vi "Main.vi"() -> ()   [LabVIEW 2020]
doc: "This Continuous Measurement sample project is based on the Queued Message Handler template.\n\nThe Event Handling Loop generates messages based on user interface actions.\n\nThe Message Handling Loop processes messages generated by the Event Handling Loop, or by other messages. There are also Acquisition and Logging message handling loop subVIs, and a chart updating loop.\n\n20190717\nIntégration de la classe Image acquisition \nIntégration de la classe CAMERA_IDS\n\nModification de la FIFO, elle est limitée à 4096 image ; \nacquisition se fait en fonction de la fréquence trame ; \naprès la sauvegarde des images on repasse à l'état acquisition. \n\n20170719\nIntegration de la classe camera PCO.\nLa fonction RUN est deplace dans getImage, pour mettre la camera dans l etat Run on verifie si les deux booleens Buffer0 et Buffer1 sont a Vrai. Start met ces deux booleens a Vrai ensuite l4un est le complement de l autre.\nModification de l affichage de Sav\nModification de la boite de dialogue maintenant on affiche les anciennes valeurs\nModification de init et exit : \nOn fait un seul init ;\non arrete pas la camera avec Stop mais avec Exit.\nAcquisition au format U16, sauvegarde FITS au format U16\nOn ralentit l affichage des images a 10 Hz> \nTest ROI 960x960 Trigger Externe 100 Hz on arrive a acquerir des cubes de 1024 images."
uses:
  UI Data.ctl
  SETTING/Settings.ctl
  LOGGING/Logging Configuration.ctl
  ACQUISITION/HardwareConfiguration.ctl
  CLASS/Image Acquisition Class/Camera.lvclass
  MIRROR/mirror.lvclass
  SETTING/data_Display.ctl
  SETTING/data_Queue.ctl
  CLASS/simuCalc Class/simuCalc.lvclass
  D:/USERS/MONTRI/BABYDOL/LABVIEW/EXEMPLE_ARCHITECTURE/acquImageCont_Sav2FITS/CLASS/Image Acquisition Class/Camera.lvclass
  ACQUISITION/Acquisition.lvlib
  LOGGING/Logging.lvlib
  SETTING/Settings.lvlib
  USER_EVENT/User Event - Stop.lvlib
  MESSAGE_QUEUE/Message Queue.lvlib
panel:
  in  "milliseconds to wait":u32=20
  out "vectCom":cluster{"tabCdG[0]":sgl, "tabCdG[1]":sgl}(graph)
  in  "loop gain (0)":dbl min=0.0 max=1.0 step=0.01
  in  "closeLoop":bool
  in  "CenterOfGravity":bool
  out "tabCdG":cluster{"tabCdG[0]":sgl, "tabCdG[1]":sgl}(graph)
  in  "threshold":bool
  in  "thresholdValue (85)":dbl
  in  "Settings":bool
  in  "Save":bool
  in  "Background":bool
  in  "LUT":bool
  in  "subtract Backgound":bool
  out "Data":sgl[][](graph)
  out "Status":string
  in  "Start":bool
  in  "Stop":bool
  in  "Exit":bool
  # "Continuous Image Acquisition"
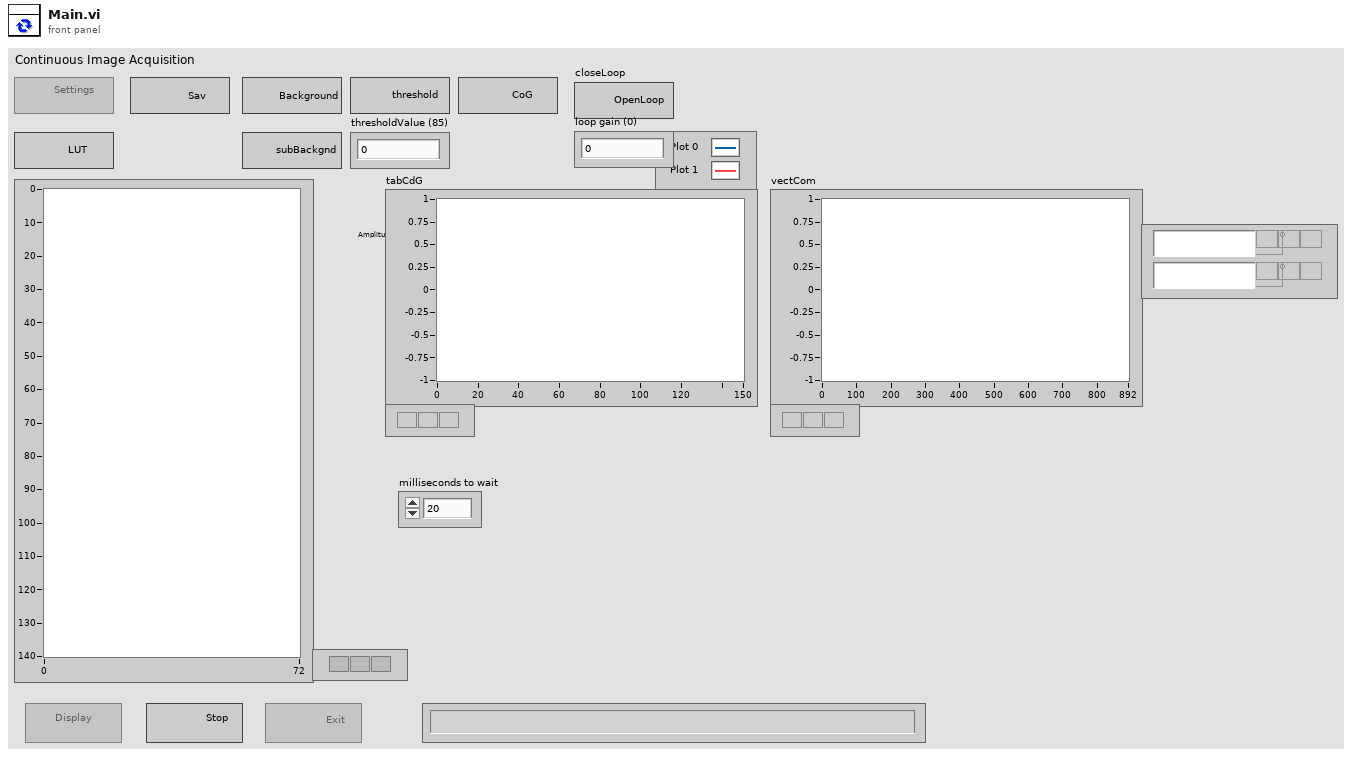
[diagram p1: front panel]
types:
  T1 = typedef "data_Queue.ctl" = cluster{"tabIma":u16[][], "tabCdG":sgl[], "vectCom":sgl[]}
  T2 = typedef "data_Display.ctl" = cluster{"tabIma":sgl[][], "tabCdG":sgl[], "vectCom":sgl[]}
  T3 = typedef "Settings.lvlib/Settings.ctl" = cluster{"Logging Configuration":T4, "camera":T5}
  T4 = typedef "Logging.lvlib/Logging Configuration.ctl" = cluster{"Log File Base Path":path, "NbrIma":i32}
  T5 = typedef "Acquisition.lvlib/HardwareConfiguration.ctl" = cluster{"Camera.lvclass":refnum<class "Camera.lvclass">, "InClusTiming 2":cluster{"Pixelclock":i32, "Exposure":dbl, "ExposureTimeBase":u16, "Framerate":dbl, "TriggerMode":u16}, "ROI":cluster{"PosX":i32, "PosY":i32, "Width":i32, "Height":i32}, "File Path Control":path, "mirror.lvclass":refnum<class "mirror.lvclass">}
  T6 = typedef "UI Data.ctl" = cluster{"Start Ref":refnum<vi>, "Save Ref":refnum<vi>, "Background":refnum<vi>, "Stop Ref":refnum<vi>, "Settings Ref":refnum<vi>, "Exit Ref":refnum<vi>, "Status Ref":refnum<vi>, "Data Ref":refnum<vi>}
  T7 = typedef "Message Queue.lvlib/All Message Queues.ctl" = cluster{"UI":refnum<queue>, "Acquisition":refnum<queue>, "Logging":refnum<queue>}
  T8 = cluster{"threshold":bool, "thresholdValue (0)":dbl}
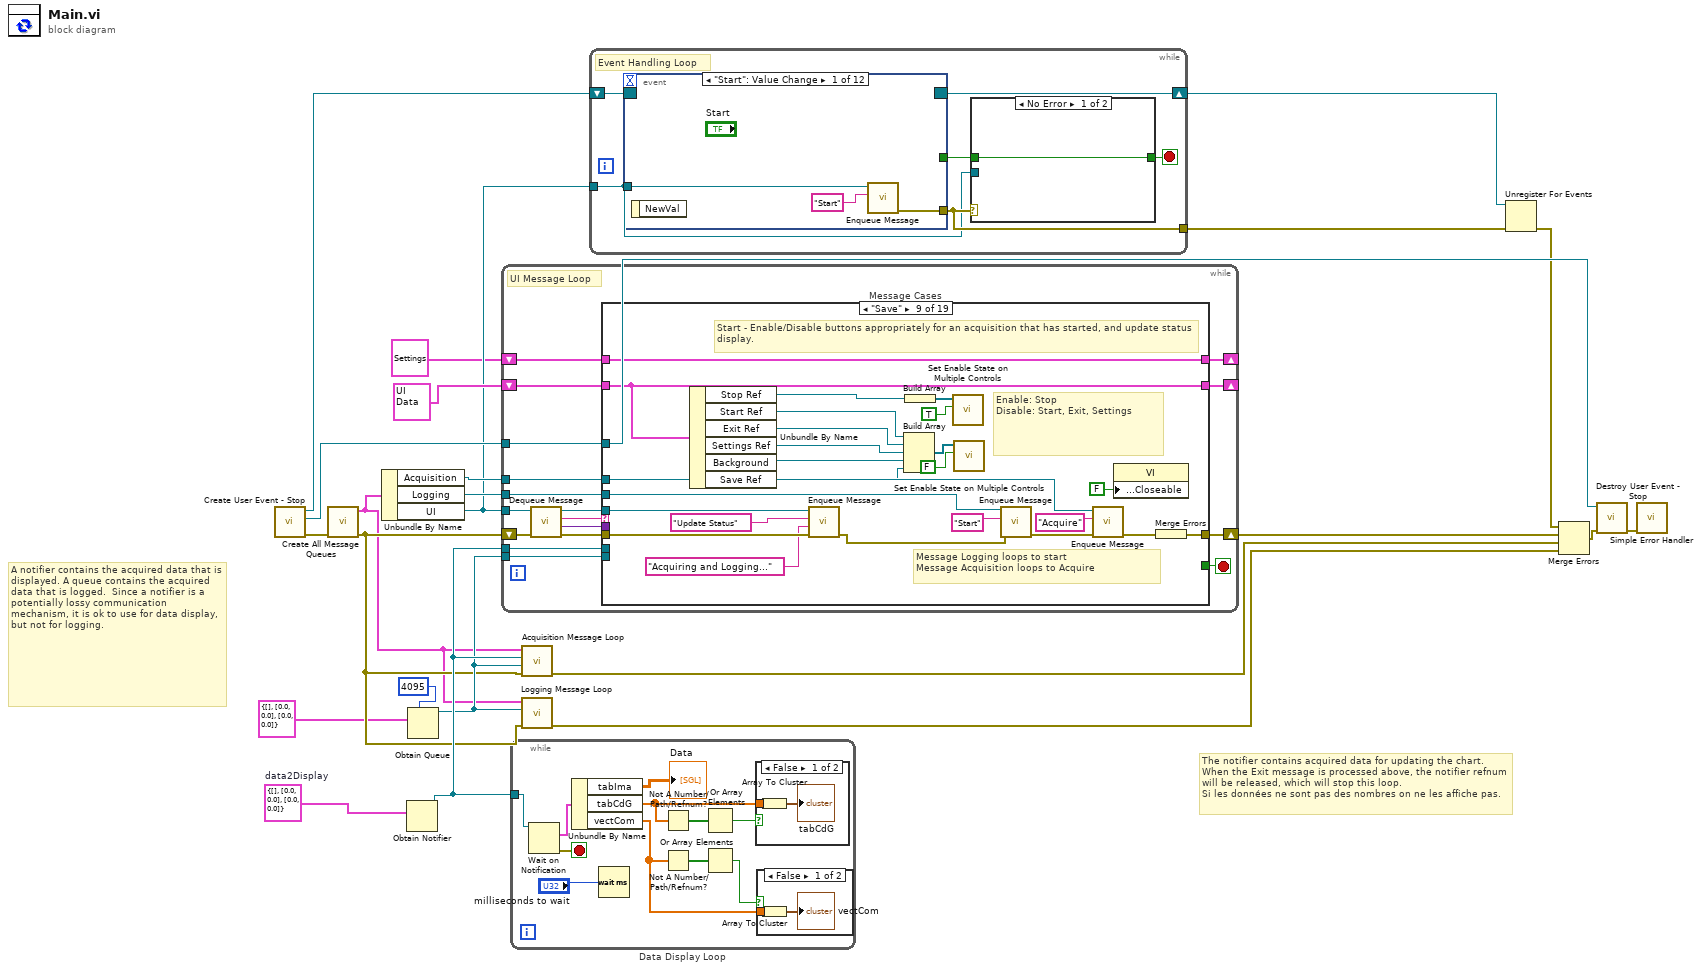
[diagram p0: block diagram]
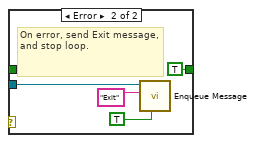
[diagram p4: hidden frame]
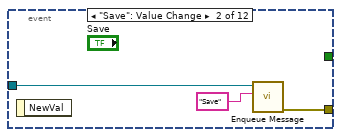
[diagram p5: hidden frame]
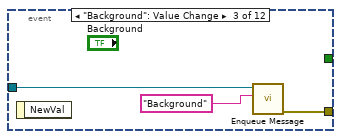
[diagram p6: hidden frame]
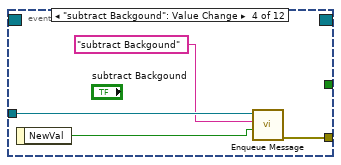
[diagram p7: hidden frame]
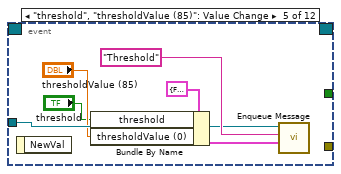
[diagram p8: hidden frame]
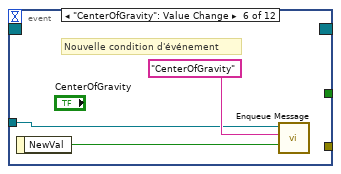
[diagram p9: hidden frame]
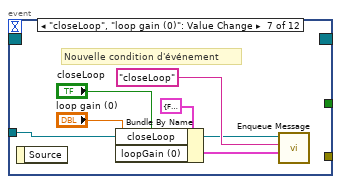
[diagram p10: hidden frame]
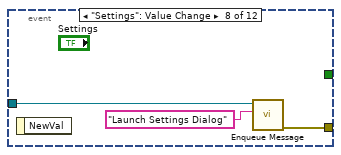
[diagram p11: hidden frame]
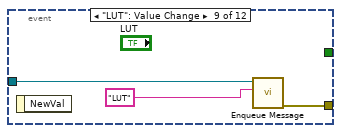
[diagram p12: hidden frame]
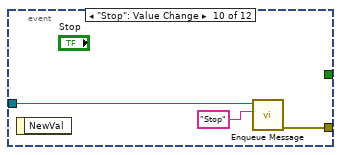
[diagram p13: hidden frame]
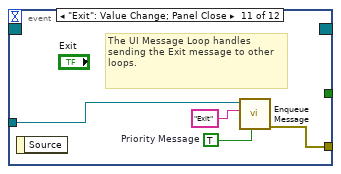
[diagram p14: hidden frame]
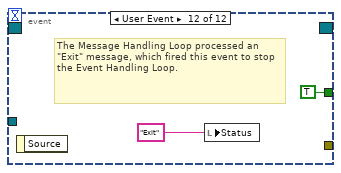
[diagram p15: hidden frame]
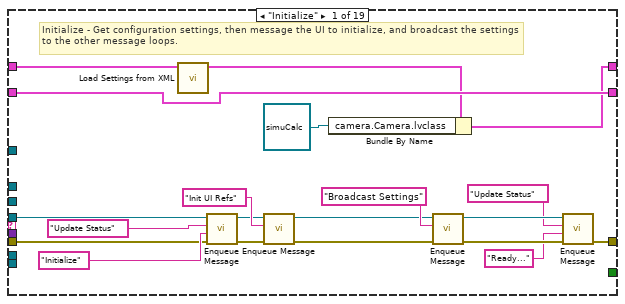
[diagram p16: hidden frame]
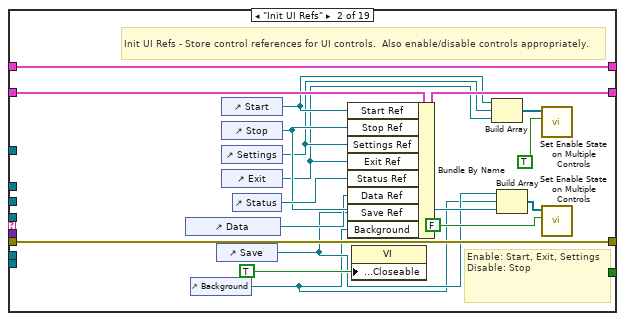
[diagram p17: hidden frame]
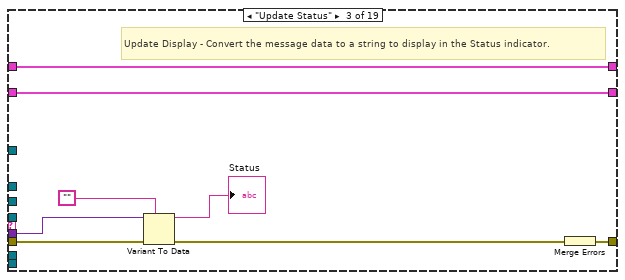
[diagram p18: hidden frame]
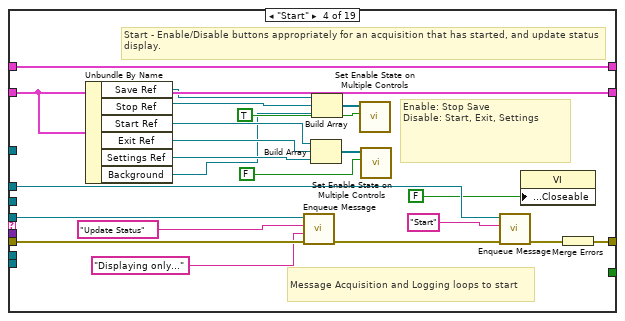
[diagram p19: hidden frame]
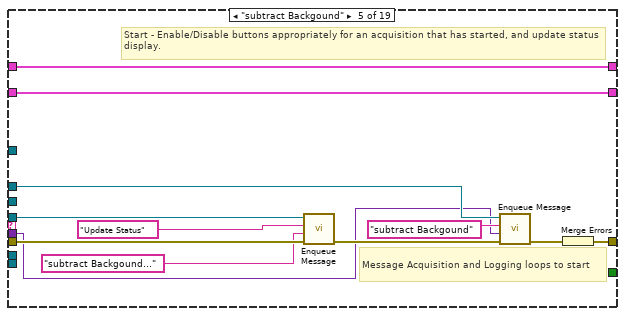
[diagram p20: hidden frame]
diagram:
  w2 = T2 {"tabIma"=[], "tabCdG"=[0.0, 0.0], "vectCom"=[0.0, 0.0]}  # data2Display
  # "A notifier contains the acquired data that is displayed. A queue contains the acquired data that is logged.  Since a notifier is a potentially lossy communication mechanism, it is ok to use for data display, but not for logging."
  # "The notifier contains acquired data for updating the chart. When the Exit message is processed above, the notifier refnum will be released, which will stop this loop.\nSi les données ne sont pas des nombres on ne les affiche pas."
  n1 = call "Create User Event - Stop.vi"() -> ("error out"=w17:errorcluster, "User Event - Stop"=w19:refnum<user-event>, "Stop Event Registration Refnum"=w20:refnum<event-registration>)  [unwired: 9 in]
  n2 = call "Create All Message Queues.vi"("error in (no error)"=w17) -> ("error out"=w4:errorcluster, "Message Queues out"=w3:T7)  [unwired: 9 in]
  n3 = Unbundle By Name(w3) -> ("Acquisition"=w12:refnum<queue>, "Logging"=w11:refnum<queue>, "UI"=w10:refnum<queue>)
  n4 = Obtain Notifier(notification data type=w2) -> (notifier out=w8:refnum<notifier>)  [unwired: 3 in, 2 out]
  n5 = Obtain Queue(max queue size (-1, unlimited)=4095, element data type=T1 {"tabIma"=[], "tabCdG"=[0.0, 0.0], "vectCom"=[0.0, 0.0]} ("Cluster")) -> (queue out=w7:refnum<queue>)  [unwired: 3 in, 2 out]
  n6 = while {
    tunnel: w10 -> [w32]
    tunnel: w19 -> [w38]
    shift-right: [w39] -> w23
    shift-left: w4 -> [w37]
    shift-right: [w31] -> _
    shift-left: T3 {"Logging Configuration"={"Log File Base Path"=path "F:/DATA/test.fits", "NbrIma"=1}, "camera"={"Camera.lvclass"=refnum, "InClusTiming 2"={"Pixelclock"=0, "Exposure"=0.0, "ExposureTimeBase"=0, "Framerate"=0.0, "TriggerMode"=0}, "ROI"={"PosX"=0, "PosY"=0, "Width"=0, "Height"=0}, "File Path Control"=path "", "mirror.lvclass"=refnum}} ("Settings") -> [w30]
    shift-right: [w28] -> _
    shift-left: T6 {"Start Ref"=refnum, "Save Ref"=refnum, "Background"=refnum, "Stop Ref"=refnum, "Settings Ref"=refnum, "Exit Ref"=refnum, "Status Ref"=refnum, "Data Ref"=refnum} ("Measurement UI Controls") -> [w29]
    tunnel: w12 -> [w27]
    tunnel: w11 -> [w26]
    tunnel: w8 -> [w25]
    tunnel: w7 -> [w24]
    stop <- w40 stop-if-true
    # "UI Message Loop"
    n7 = call "Dequeue Message.vi"("error in (no error)"=w37, "Message Queue"=w32) -> ("error out"=w36:errorcluster, "Message Data"=w34:variant, "Message"=w35:string, "dup Message Queue"=w33:refnum<queue>)  [unwired: 6 in]
    n8 = case "Message Cases" shown="\"Save\"" w35 {
      selector: w35 -> [_ _ _ _ _ _ _ _ _ _ _ _ _ _ _ _ _ _ w316]
      tunnel: w33 -> [w44 _ _ w106 w118 w130 w142 w154 w179 w204 w226 _ w243 w257 _ _ w292 w305 _]
      tunnel: w36 -> [w45 w77 w84 w105 w117 w129 w141 w153 w178 w203 w225 w233 w245 w265 w271 w272 w294 w306 _]
      tunnel: [w57 w77 w85 w107 w119 w131 w143 w155 w180 w205 w227 w238 w240 w266 w270 w276 w298 w310 w314] -> w39
      tunnel: [_ _ _ _ _ _ _ _ _ _ _ _ _ TRUE _ _ _ _ _] -> w40
      tunnel: w34 -> [_ _ w83 _ w108 w120 w132 w144 _ _ _ _ _ _ _ _ _ _ _]
      tunnel: w38 -> [_ _ _ _ _ _ _ _ _ _ _ _ _ w264 _ _ _ _ _]
      tunnel: [w48 w76 w79 w104 w116 w128 w140 w152 w177 w202 w224 w236 w242 w262 w269 w275 w297 w309 w312] -> w31
      tunnel: w30 -> [w60 w76 w79 w104 w116 w128 w140 w152 w177 w202 w224 w236 w246 w262 w269 w275 w297 w309 w312]
      tunnel: w29 -> [w53 w75 w78 w101 w113 w125 w137 w149 w174 w199 w221 w231 w239 w260 w268 w274 w289 w302 w311]
      tunnel: [w53 w73 w78 w101 w113 w125 w137 w149 w174 w199 w221 w231 w239 w260 w268 w274 w289 w302 w311] -> w28
      tunnel: w27 -> [_ _ _ w91 w111 w123 w135 w147 w159 w184 w211 w230 _ w259 _ _ _ _ _]
      tunnel: w26 -> [_ _ _ _ _ _ _ _ w164 w189 _ w229 _ w258 _ _ _ _ _]
      tunnel: w25 -> [_ _ _ _ _ _ _ _ _ _ _ _ _ w256 _ _ _ _ _]
      tunnel: w24 -> [_ _ _ _ _ _ _ _ _ _ _ _ _ w252 _ _ _ _ _]
      frame "Initialize" {
        # "Initialize - Get configuration settings, then message the UI to initialize, and broadcast the settings to the other message loops."
        n9 = call "Load Settings from XML.vi"("Settings in"=w60) -> ("Settings out"=w49:T3)  [unwired: 9 in, 1 out]
        n10 = call "Enqueue Message.vi"("error in (no error)"=w45, "Message Data"="Initialize" ("Acquiring and Logging..."), "Message"="Update Status", "Message Queue"=w44) -> ("error out"=w43:errorcluster, "dup Message Queue"=w42:refnum<queue>)  [unwired: 6 in]
        n11 = call "Enqueue Message.vi"("error in (no error)"=w43, "Message"="Init UI Refs", "Message Queue"=w42) -> ("error out"=w50:errorcluster, "dup Message Queue"=w51:refnum<queue>)  [unwired: 7 in]
        n12 = Bundle By Name(cluster=w49, "camera.Camera.lvclass"=refnum<class "simuCalc.lvclass"> refnum ("simuCalc.lvclass")) -> (w48:T3)
        n13 = call "Enqueue Message.vi"("error in (no error)"=w50, "Message"="Broadcast Settings", "Message Queue"=w51) -> ("error out"=w59:errorcluster, "dup Message Queue"=w58:refnum<queue>)  [unwired: 7 in]
        n14 = call "Enqueue Message.vi"("error in (no error)"=w59, "Message Data"="Ready..." ("Ready..."), "Message"="Update Status", "Message Queue"=w58) -> ("error out"=w57:errorcluster)  [unwired: 6 in, 1 out]
      }
      frame "Init UI Refs" {
        # "Enable: Start, Exit, Settings\nDisable: Stop"
        # "Init UI Refs - Store control references for UI controls.  Also enable/disable controls appropriately."
        n15 = control-ref of="Data"() -> (w63:refnum<vi>)
        n16 = control-ref of="Background"() -> (w61:refnum<vi>)
        n17 = control-ref of="Save"() -> (w62:refnum<vi>)
        n18 = control-ref of="Start"() -> (w67:refnum<vi>)
        n19 = control-ref of="Stop"() -> (w68:refnum<vi>)
        n20 = control-ref of="Settings"() -> (w66:refnum<vi>)
        n21 = control-ref of="Exit"() -> (w65:refnum<vi>)
        n22 = control-ref of="Status"() -> (w74:refnum<vi>)
        n23 = Bundle By Name(cluster=w75, "Start Ref"=w67, "Stop Ref"=w68, "Settings Ref"=w66, "Exit Ref"=w65, "Status Ref"=w74, "Data Ref"=w63, "Save Ref"=w62, "Background"=w61) -> (w73:T6)
        n24 = property class="VI"("Front Panel.Closeable"=TRUE ("Front Panel Window:Closeable")) -> ()  [unwired: 2 in, 2 out]
        n25 = Build Array(w67, w66, w65) -> (w71:refnum<vi>[])
        n26 = Build Array(w62, w61, w68) -> (w70:refnum<vi>[])
        n27 = call "Set Enable State on Multiple Controls.vi"("Enable?"=TRUE, "Controls"=w71) -> ()  [unwired: 10 in]
        n28 = call "Set Enable State on Multiple Controls.vi"("Enable?"=FALSE, "Controls"=w70) -> ()  [unwired: 10 in]
      }
      frame "Update Status" {
        # "Update Display - Convert the message data to a string to display in the Status indicator."
        n29 = Variant To Data(error in=w84, type="", Variant=w83) -> (data=→"Status":string, error out=w81:errorcluster)
        n30 = Merge Errors(w81) -> (w85:errorcluster)
      }
      frame "Start" {
        # "Message Acquisition and Logging loops to start"
        # "Enable: Stop Save\nDisable: Start, Exit, Settings"
        # "Start - Enable/Disable buttons appropriately for an acquisition that has started, and update status display."
        n31 = Unbundle By Name(w101) -> ("Save Ref"=w87:refnum<vi>, "Stop Ref"=w96:refnum<vi>, "Start Ref"=w95:refnum<vi>, "Exit Ref"=w94:refnum<vi>, "Settings Ref"=w93:refnum<vi>, "Background"=w86:refnum<vi>)
        n32 = call "Enqueue Message.vi"("error in (no error)"=w105, "Message Data"="Displaying only..." ("Acquiring and Logging..."), "Message"="Update Status", "Message Queue"=w106) -> ("error out"=w88:errorcluster)  [unwired: 6 in, 1 out]
        n33 = Build Array(w95, w94, w93) -> (w99:refnum<vi>[])
        n34 = Build Array(w87, w96, w86) -> (w98:refnum<vi>[])
        n35 = call "Set Enable State on Multiple Controls.vi"("Enable?"=TRUE, "Controls"=w98) -> ()  [unwired: 10 in]
        n36 = call "Set Enable State on Multiple Controls.vi"("Enable?"=FALSE, "Controls"=w99) -> ()  [unwired: 10 in]
        n37 = call "Enqueue Message.vi"("error in (no error)"=w88, "Message"="Start", "Message Queue"=w91) -> ("error out"=w92:errorcluster)  [unwired: 7 in, 1 out]
        n38 = property class="VI"("Front Panel.Closeable"=FALSE ("Front Panel Window:Closeable")) -> ()  [unwired: 2 in, 2 out]
        n39 = Merge Errors(w92) -> (w107:errorcluster)
      }
      frame "subtract Backgound" {
        # "Message Acquisition and Logging loops to start"
        # "Start - Enable/Disable buttons appropriately for an acquisition that has started, and update status display."
        n40 = call "Enqueue Message.vi"("error in (no error)"=w117, "Message Data"="subtract Backgound..." ("Acquiring and Logging..."), "Message"="Update Status", "Message Queue"=w118) -> ("error out"=w109:errorcluster)  [unwired: 6 in, 1 out]
        n41 = call "Enqueue Message.vi"("error in (no error)"=w109, "Message Data"=w108, "Message"="subtract Backgound", "Message Queue"=w111) -> ("error out"=w112:errorcluster)  [unwired: 6 in, 1 out]
        n42 = Merge Errors(w112) -> (w119:errorcluster)
      }
      frame "Threshold" {
        # "Message Acquisition and Logging loops to start"
        # "Start - Enable/Disable buttons appropriately for an acquisition that has started, and update status display."
        n43 = call "Enqueue Message.vi"("error in (no error)"=w129, "Message Data"="Threshold..." ("Acquiring and Logging..."), "Message"="Update Status", "Message Queue"=w130) -> ("error out"=w121:errorcluster)  [unwired: 6 in, 1 out]
        n44 = call "Enqueue Message.vi"("error in (no error)"=w121, "Message Data"=w120, "Message"="Threshold", "Message Queue"=w123) -> ("error out"=w124:errorcluster)  [unwired: 6 in, 1 out]
        n45 = Merge Errors(w124) -> (w131:errorcluster)
      }
      frame "CenterOfGravity" {
        # "Message Acquisition and Logging loops to start"
        # "Start - Enable/Disable buttons appropriately for an acquisition that has started, and update status display."
        n46 = call "Enqueue Message.vi"("error in (no error)"=w141, "Message Data"="CenterOfGravity...." ("Acquiring and Logging..."), "Message"="Update Status", "Message Queue"=w142) -> ("error out"=w133:errorcluster)  [unwired: 6 in, 1 out]
        n47 = call "Enqueue Message.vi"("error in (no error)"=w133, "Message Data"=w132, "Message"="CenterOfGravity", "Message Queue"=w135) -> ("error out"=w136:errorcluster)  [unwired: 6 in, 1 out]
        n48 = Merge Errors(w136) -> (w143:errorcluster)
      }
      frame "closeLoop" {
        # "Message Acquisition and Logging loops to start"
        # "Start - Enable/Disable buttons appropriately for an acquisition that has started, and update status display."
        n49 = call "Enqueue Message.vi"("error in (no error)"=w153, "Message Data"="closeLoop...." ("Acquiring and Logging..."), "Message"="Update Status", "Message Queue"=w154) -> ("error out"=w145:errorcluster)  [unwired: 6 in, 1 out]
        n50 = call "Enqueue Message.vi"("error in (no error)"=w145, "Message Data"=w144, "Message"="closeLoop", "Message Queue"=w147) -> ("error out"=w148:errorcluster)  [unwired: 6 in, 1 out]
        n51 = Merge Errors(w148) -> (w155:errorcluster)
      }
      frame "Save" {
        # "Message Logging loops to start\nMessage Acquisition loops to Acquire"
        # "Enable: Stop\nDisable: Start, Exit, Settings"
        # "Start - Enable/Disable buttons appropriately for an acquisition that has started, and update status display."
        n52 = Unbundle By Name(w174) -> ("Stop Ref"=w169:refnum<vi>, "Start Ref"=w168:refnum<vi>, "Exit Ref"=w167:refnum<vi>, "Settings Ref"=w166:refnum<vi>, "Background"=w157:refnum<vi>, "Save Ref"=w156:refnum<vi>)
        n53 = call "Enqueue Message.vi"("error in (no error)"=w178, "Message Data"="Acquiring and Logging..." ("Acquiring and Logging..."), "Message"="Update Status", "Message Queue"=w179) -> ("error out"=w158:errorcluster)  [unwired: 6 in, 1 out]
        n54 = Build Array(w168, w167, w166, w157, w156) -> (w172:refnum<vi>[])
        n55 = Build Array(w169) -> (w171:refnum<vi>[])
        n56 = call "Set Enable State on Multiple Controls.vi"("Enable?"=TRUE, "Controls"=w171) -> ()  [unwired: 10 in]
        n57 = call "Set Enable State on Multiple Controls.vi"("Enable?"=FALSE, "Controls"=w172) -> ()  [unwired: 10 in]
        n58 = call "Enqueue Message.vi"("error in (no error)"=w158, "Message"="Start", "Message Queue"=w164) -> ("error out"=w163:errorcluster)  [unwired: 7 in, 1 out]
        n59 = call "Enqueue Message.vi"("error in (no error)"=w163, "Message"="Acquire", "Message Queue"=w159) -> ("error out"=w162:errorcluster)  [unwired: 7 in, 1 out]
        n60 = property class="VI"("Front Panel.Closeable"=FALSE ("Front Panel Window:Closeable")) -> ()  [unwired: 2 in, 2 out]
        n61 = Merge Errors(w162) -> (w180:errorcluster)
      }
      frame "Background" {
        # "Message Logging loops to start\nMessage Acquisition loops to Acquire"
        # "Enable: Stop\nDisable: Start, Exit, Settings"
        # "Start - Enable/Disable buttons appropriately for an acquisition that has started, and update status display."
        n62 = Unbundle By Name(w199) -> ("Stop Ref"=w194:refnum<vi>, "Start Ref"=w193:refnum<vi>, "Exit Ref"=w192:refnum<vi>, "Settings Ref"=w191:refnum<vi>, "Save Ref"=w182:refnum<vi>, "Background"=w181:refnum<vi>)
        n63 = call "Enqueue Message.vi"("error in (no error)"=w203, "Message Data"="Acquiring Background..." ("Acquiring and Logging..."), "Message"="Update Status", "Message Queue"=w204) -> ("error out"=w183:errorcluster)  [unwired: 6 in, 1 out]
        n64 = Build Array(w193, w192, w191, w182, w181) -> (w197:refnum<vi>[])
        n65 = Build Array(w194) -> (w196:refnum<vi>[])
        n66 = call "Set Enable State on Multiple Controls.vi"("Enable?"=TRUE, "Controls"=w196) -> ()  [unwired: 10 in]
        n67 = call "Set Enable State on Multiple Controls.vi"("Enable?"=FALSE, "Controls"=w197) -> ()  [unwired: 10 in]
        n68 = call "Enqueue Message.vi"("error in (no error)"=w183, "Message"="StartBackground", "Message Queue"=w189) -> ("error out"=w188:errorcluster)  [unwired: 7 in, 1 out]
        n69 = call "Enqueue Message.vi"("error in (no error)"=w188, "Message"="Acquire", "Message Queue"=w184) -> ("error out"=w187:errorcluster)  [unwired: 7 in, 1 out]
        n70 = property class="VI"("Front Panel.Closeable"=FALSE ("Front Panel Window:Closeable")) -> ()  [unwired: 2 in, 2 out]
        n71 = Merge Errors(w187) -> (w205:errorcluster)
      }
      frame "Stop" {
        # "Message Acquisition and Logging loops to stop"
        # "Enable: Start, Exit, Settings\nDisable: Stop"
        # "Stop - Enable/Disable buttons appropriately for an acquisition that has stopped, and update status display."
        n72 = Unbundle By Name(w221) -> ("Save Ref"=w207:refnum<vi>, "Stop Ref"=w216:refnum<vi>, "Start Ref"=w215:refnum<vi>, "Exit Ref"=w214:refnum<vi>, "Settings Ref"=w213:refnum<vi>, "Exit Ref"=w206:refnum<vi>)
        n73 = call "Enqueue Message.vi"("error in (no error)"=w225, "Message Data"="Ready..." ("Ready..."), "Message"="Update Status", "Message Queue"=w226) -> ("error out"=w208:errorcluster)  [unwired: 6 in, 1 out]
        n74 = Build Array(w215, w214, w213, w206) -> (w219:refnum<vi>[])
        n75 = Build Array(w207, w216) -> (w218:refnum<vi>[])
        n76 = call "Set Enable State on Multiple Controls.vi"("Enable?"=FALSE, "Controls"=w218) -> ()  [unwired: 10 in]
        n77 = call "Set Enable State on Multiple Controls.vi"("Enable?"=TRUE, "Controls"=w219) -> ()  [unwired: 10 in]
        n78 = call "Enqueue Message.vi"("error in (no error)"=w208, "Message"="Stop", "Message Queue"=w211) -> ("error out"=w212:errorcluster)  [unwired: 7 in, 1 out]
        n79 = property class="VI"("Front Panel.Closeable"=TRUE ("Front Panel Window:Closeable")) -> ()  [unwired: 2 in, 2 out]
        n80 = Merge Errors(w212) -> (w227:errorcluster)
      }
      frame "Broadcast settings" {
        w232 = "Update Settings" ("Message")
        # "Send the 'Update Settings' message to the Logging and Acqusition message loops."
        n81 = Unbundle By Name(w236) -> ("camera"=w228:T5, "Logging Configuration"=w235:T4)
        n82 = call "Enqueue Message.vi"("Message Data"=w228, "Message"=w232, "Message Queue"=w230) -> ("error out"=w237:errorcluster)  [unwired: 7 in, 1 out]
        n83 = call "Enqueue Message.vi"("error in (no error)"=w237, "Message Data"=w235, "Message"=w232, "Message Queue"=w229) -> ("error out"=w234:errorcluster)  [unwired: 6 in, 1 out]
        n84 = Merge Errors(w234, w233) -> (w238:errorcluster)
      }
      frame "Launch Settings Dialog" {
        # "Launch the Settings Dialog when the user clicks the 'Settings' button."
        n85 = call "Settings Dialog.vi"("error in (no error)"=w245, "Settings in"=w246) -> ("error out"=w241:errorcluster, "Cancelled?"=w244:bool, "Settings out"=w242:T3)  [unwired: 6 in, 1 out]
        n86 = case shown="False" w244 {
          tunnel: w243 -> [w250 _]
          tunnel: w241 -> [w249 w251]
          tunnel: [w248 w251] -> w240
          frame False {
            n87 = call "Enqueue Message.vi"("error in (no error)"=w249, "Message"="Broadcast Settings", "Message Queue"=w250) -> ("error out"=w248:errorcluster)  [unwired: 7 in, 1 out]
          }
          frame True {
          }
        }
      }
      frame "Exit" {
        w261 = "Exit" ("Message")
        # "Don't check the error outs. The acquisition and logging queues may have already been released."
        # "Close references owned by the Main VI."
        # "Stop the VI"
        # "Exit - Fire the User Event to stop the Event Handling Loop.  Also send Exit messages to the Acqusition and Logging loops."
        n88 = Release Queue(queue=w257, error in (no error)=w265) -> (error out=w255:errorcluster)  [unwired: 1 in, 2 out]
        n89 = call "Fire User Event - Stop.vi"("User Event - Stop"=w264) -> ("error out"=w263:errorcluster)  [unwired: 10 in]
        n90 = Release Notifier(notifier=w256, error in (no error)=w255) -> (error out=w254:errorcluster)  [unwired: 1 in, 2 out]
        n91 = Release Queue(queue=w252, error in (no error)=w254) -> (error out=w253:errorcluster)  [unwired: 1 in, 2 out]
        n92 = call "Enqueue Message.vi"("Message"=w261, "Message Queue"=w259) -> ()  [unwired: 8 in, 2 out]
        n93 = call "Enqueue Message.vi"("Message"=w261, "Message Queue"=w258) -> ()  [unwired: 8 in, 2 out]
        n94 = Merge Errors(w263, w253) -> (w266:errorcluster)
      }
      frame "---Copy This Frame---" {
        # "Duplicate this frame when creating new messages.  Change this comment in the duplicated frame to describe this message."
        n95 = Merge Errors(w271) -> (w270:errorcluster)
      }
      frame "LUT" {
        # "Duplicate this frame when creating new messages.  Change this comment in the duplicated frame to describe this message."
        n96 = case shown="No Error" w272 {
          selector: w272 -> [w281 w286]
          tunnel: [w280 w286] -> w273
          frame No Error {
            n97 = Current VI's Path() -> (path=w278:path)
            n98 = call "LectFicLUT_IDL.vi"("CheminFichierLUT"=w278) -> ("TabValLUT"=w277:u32[])  [unwired: 1 out]
            n99 = Empty Array?(array=w277) -> (empty?=w279:bool)
            n100 = case shown="False" w279 {
              tunnel: w281 -> [w284 w285]
              tunnel: [w283 w285] -> w280
              tunnel: w277 -> [w282 _]
              frame False {
                n101 = property on="Data" class="IntGraph (strict)"(error in=w284, "Color Table"=w282) -> (error out=w283:errorcluster)  [unwired: 1 in, 1 out]
              }
              frame True {
              }
            }
          }
          frame Error {
          }
        }
        n102 = Merge Errors(w273) -> (w276:errorcluster)
      }
      frame "Data loged" {
        # "Duplicate this frame when creating new messages.  Change this comment in the duplicated frame to describe this message."
        n103 = Unbundle By Name(w289) -> ("Save Ref"=w288:refnum<vi>, "Background"=w287:refnum<vi>)
        n104 = Build Array(w288, w287) -> (w291:refnum<vi>[])
        n105 = call "Set Enable State on Multiple Controls.vi"("Enable?"=TRUE, "Controls"=w291) -> ()  [unwired: 10 in]
        n106 = call "Enqueue Message.vi"("error in (no error)"=w294, "Message Data"="Displaying only..." ("Acquiring and Logging..."), "Message"="Update Status", "Message Queue"=w292) -> ("error out"=w293:errorcluster)  [unwired: 6 in, 1 out]
        n107 = Merge Errors(w293) -> (w298:errorcluster)
      }
      frame "Background loged" {
        # "Duplicate this frame when creating new messages.  Change this comment in the duplicated frame to describe this message."
        n108 = Unbundle By Name(w302) -> ("Save Ref"=w301:refnum<vi>, "Background"=w300:refnum<vi>)
        n109 = Build Array(w301, w300) -> (w304:refnum<vi>[])
        n110 = call "Set Enable State on Multiple Controls.vi"("Enable?"=TRUE, "Controls"=w304) -> ()  [unwired: 10 in]
        n111 = call "Enqueue Message.vi"("error in (no error)"=w306, "Message Data"="Displaying only..." ("Acquiring and Logging..."), "Message"="Update Status", "Message Queue"=w305) -> ("error out"=w299:errorcluster)  [unwired: 6 in, 1 out]
        n112 = Merge Errors(w299) -> (w310:errorcluster)
      }
      frame Default {
        # "'Default' case only runs if there is a message that isn't defined in any of the other cases.  Output a programming error."
        n113 = Format Into String(format string="The invalid message string \"%s\" was received in the Message Handling Loop." ("Invalid Message Loop Message"), w316) -> (resulting string=w313:string)  [unwired: 2 in, 1 out]
        n114 = call <vilib>:"Error Cluster From Error Code.vi"("error message (\"\")"=w313, "error code (0)"=1) -> ("error out"=w314:errorcluster)  [unwired: 7 in]
      }
    }
  }
  n115 = while "Data Display Loop" {
    tunnel: w8 -> [w328]
    stop <- w327 stop-if-true
    n116 = Wait on Notification(notifier=w328) -> (notification=w326:T2, error out=w327:errorcluster)  [unwired: 3 in, 2 out]
    n117 = Unbundle By Name(w326) -> ("tabIma"=→"Data":sgl[][], "tabCdG"=w323:sgl[], "vectCom"=w322:sgl[])
    n118 = Wait (ms)(milliseconds to wait="milliseconds to wait") -> ()  [unwired: 1 out]
    n119 = Not A Number/Path/Refnum?(number/path/refnum=w323) -> (NaN/Path/Refnum?=w321:bool[])
    n120 = Not A Number/Path/Refnum?(number/path/refnum=w322) -> (NaN/Path/Refnum?=w320:bool[])
    n121 = Or Array Elements(Boolean array=w321) -> (logical OR=w318:bool)
    n122 = Or Array Elements(Boolean array=w320) -> (logical OR=w319:bool)
    n123 = case shown="False" w318 {
      tunnel: w323 -> [w331 _]
      frame False {
        n124 = Array To Cluster(array=w331) -> (cluster=→"tabCdG":cluster{"tabCdG[0]":sgl, "tabCdG[1]":sgl})
      }
      frame True {
      }
    }
    n125 = case shown="False" w319 {
      tunnel: w322 -> [w329 _]
      frame False {
        n126 = Array To Cluster(array=w329) -> (cluster=→"vectCom":cluster{"vectCom[0]":sgl, "vectCom[1]":sgl})
      }
      frame True {
      }
    }
  }
  n127 = call "Acquisition Message Loop.vi"("error in (no error)"=w4, "Data Queue"=w7, "Data Notifier"=w8, "Message Queues"=w3) -> ("error out"=w18:errorcluster)  [unwired: 7 in]
  n128 = call "Logging Message Loop.vi"("error in (no error)"=w4, "Data Queue"=w7, "Message Queues"=w3) -> ("error out"=w16:errorcluster)  [unwired: 8 in]
  n129 = while {
    tunnel: w10 -> [w334]
    tunnel: [w336] -> w22
    shift-right: [w333] -> w14
    shift-left: w20 -> [w335]
    stop <- w337 stop-if-true
    # "Event Handling Loop"
    n130 = event shown="[0] \"Start\": Value Change" {
      selector: w335 -> [_ _ _ _ _ _ _ _ _ _ _ _]
      dyn-events: [_ _ _ _ _ _ _ _ _ _ _ _] -> w333
      timeout: _ -> [_ _ _ _ _ _ _ _ _ _ _ _]
      tunnel: [_ _ _ _ _ _ _ _ _ _ _ TRUE ("Discard?")] -> w338
      tunnel: w334 -> [w344 w347 w350 w355 w361 w364 w370 w372 w375 w379 w381 _]
      tunnel: [w346 w349 w352 w356 _ _ _ w374 w377 w378 w384 _] -> w336
      event "Start": Value Change {
        n131 = event-data() -> ()  [unwired: 1 in, 1 out]
        n132 = call "Enqueue Message.vi"("Message"="Start", "Message Queue"=w344) -> ("error out"=w346:errorcluster)  [unwired: 8 in, 1 out]
      }
      event "Save": Value Change {
        n133 = event-data() -> ()  [unwired: 1 in, 1 out]
        n134 = call "Enqueue Message.vi"("Message"="Save", "Message Queue"=w347) -> ("error out"=w349:errorcluster)  [unwired: 8 in, 1 out]
      }
      event "Background": Value Change {
        n135 = event-data() -> ()  [unwired: 1 in, 1 out]
        n136 = call "Enqueue Message.vi"("Message"="Background", "Message Queue"=w350) -> ("error out"=w352:errorcluster)  [unwired: 8 in, 1 out]
      }
      event "subtract Backgound": Value Change {
        n137 = event-data() -> ("NewVal"=w354:bool)  [unwired: 1 in]
        n138 = call "Enqueue Message.vi"("Message Data"=w354, "Message"="subtract Backgound", "Message Queue"=w355) -> ("error out"=w356:errorcluster)  [unwired: 7 in, 1 out]
      }
      event "threshold", "thresholdValue (85)": Value Change {
        n139 = event-data() -> ()  [unwired: 1 in, 1 out]
        n140 = Bundle By Name(cluster=T8 {"threshold"=FALSE, "thresholdValue (0)"=0.0}, "threshold"="threshold", "thresholdValue (0)"="thresholdValue (85)") -> (w358:T8)
        n141 = call "Enqueue Message.vi"("Message Data"=w358, "Message"="Threshold", "Message Queue"=w361) -> ()  [unwired: 7 in, 2 out]
      }
      event "CenterOfGravity": Value Change {
        # "Nouvelle condition d'événement"
        n142 = event-data() -> ("NewVal"=w363:bool)  [unwired: 1 in]
        n143 = call "Enqueue Message.vi"("Message Data"=w363, "Message"="CenterOfGravity", "Message Queue"=w364) -> ()  [unwired: 7 in, 2 out]
      }
      event "closeLoop", "loop gain (0)": Value Change {
        # "Nouvelle condition d'événement"
        n144 = event-data() -> ()  [unwired: 1 in, 1 out]
        n145 = Bundle By Name(cluster=cluster{"closeLoop":bool, "loopGain (0)":dbl} {"closeLoop"=FALSE, "loopGain (0)"=0.0}, "closeLoop"="closeLoop", "loopGain (0)"="loop gain (0)") -> (w369:cluster{"closeLoop":bool, "loopGain (0)":dbl})
        n146 = call "Enqueue Message.vi"("Message Data"=w369, "Message"="closeLoop", "Message Queue"=w370) -> ()  [unwired: 7 in, 2 out]
      }
      event "Settings": Value Change {
        n147 = event-data() -> ()  [unwired: 1 in, 1 out]
        n148 = call "Enqueue Message.vi"("Message"="Launch Settings Dialog", "Message Queue"=w372) -> ("error out"=w374:errorcluster)  [unwired: 8 in, 1 out]
      }
      event "LUT": Value Change {
        n149 = event-data() -> ()  [unwired: 1 in, 1 out]
        n150 = call "Enqueue Message.vi"("Message"="LUT", "Message Queue"=w375) -> ("error out"=w377:errorcluster)  [unwired: 8 in, 1 out]
      }
      event "Stop": Value Change {
        n151 = event-data() -> ()  [unwired: 1 in, 1 out]
        n152 = call "Enqueue Message.vi"("Message"="Stop", "Message Queue"=w379) -> ("error out"=w378:errorcluster)  [unwired: 8 in, 1 out]
      }
      event "Exit": Value Change; Panel Close {
        w382 = TRUE  # Priority Message
        # "The UI Message Loop handles sending the Exit message to other loops."
        n153 = event-data() -> ()  [unwired: 1 in, 1 out]
        n154 = call "Enqueue Message.vi"("Priority Message? (F)"=w382, "Message"="Exit", "Message Queue"=w381) -> ("error out"=w384:errorcluster)  [unwired: 7 in, 1 out]
      }
      event User Event {
        # "The Message Handling Loop processed an \"Exit\" message, which fired this event to stop the Event Handling Loop."
        n155 = event-data() -> ()  [unwired: 1 in, 1 out]
        n156 = local write "Status"("Exit" ("Exit String")) -> ()
      }
    }
    n157 = case shown="No Error" w336 {
      tunnel: [w339 TRUE ("Discard?")] -> w337
      tunnel: w338 -> [w339 _]
      tunnel: w334 -> [_ w340]
      frame No Error {
      }
      frame Error {
        # "On error, send Exit message, and stop loop."
        n158 = call "Enqueue Message.vi"("Priority Message? (F)"=TRUE ("Discard?"), "Message"="Exit", "Message Queue"=w340) -> ()  [unwired: 7 in, 2 out]
      }
    }
  }
  n159 = Unregister For Events(event registration refnum=w14, error in=w22) -> (error out=w15:errorcluster)
  n160 = Merge Errors(w15, w23, w18, w16) -> (w21:errorcluster)
  n161 = call "Destroy User Event - Stop.vi"("error in (no error)"=w21, "User Event - Stop"=w19) -> ("error out"=w9:errorcluster)  [unwired: 9 in]
  n162 = call <vilib>:"Simple Error Handler.vi"("error in (no error)"=w9) -> ()  [unwired: 4 in, 5 out]
